vi "4 DDS 16SPC.vi"(8 "input valid":bool=TRUE, 9 "pdw in":T2 {"frequency shift" format="%#_12f"}, 10 "free DDS before me?":bool, 11 "new PDW in":bool) -> (0 "output valid":bool, 1 "state of every DDS":bool[](array[boolean]), 2 "have free DDS":bool, 3 "IQ out":T1[](array[typedef]))   [LabVIEW 2022 SP3]
doc: "transmit pulse with one free DDS inside.\nmust have no DDS before him (the distribute is to give the lowest mun DDS the pulse)"
uses:
  pulse_tx_vis/pdw.ctl
  pulse_tx_vis/mode_type.ctl
  <instrlib>/_niInstr/DSP/v1/Shared/Public/IQ Data.ctl
  <instrlib>/_niInstr/DSP/v1/Shared/niInstr DSP v1 Shared.lvlib
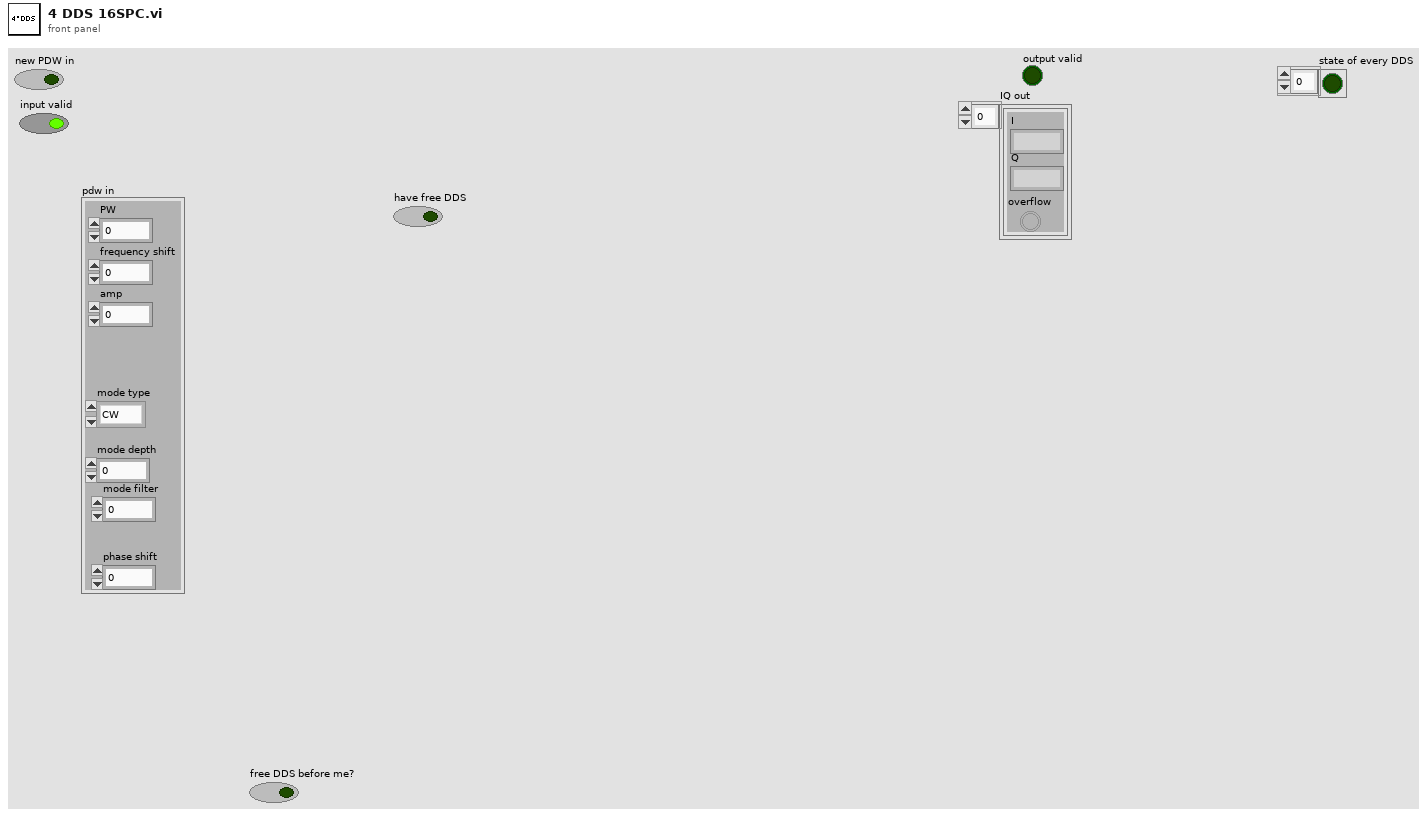
[diagram p1: front panel]
types:
  T1 = typedef "niInstr DSP v1 Shared.lvlib/IQ Data.ctl" = cluster{"I":fxp<+/-,18,1>, "Q":fxp<+/-,18,1>, "overflow":bool}
  T2 = typedef "pdw.ctl" = cluster{"PW":u32, "frequency shift":fxp<+/-,48,0>, "amp":fxp<+/-,18,1>, "mode type":T3, "mode depth":u32, "mode filter":u8, "phase shift":fxp<+/-,16,1>}
  T3 = typedef "mode_type.ctl" = enum8{"CW", "NC - CW", "NC - cw", "LFM", "BPSK", "QPSK"}
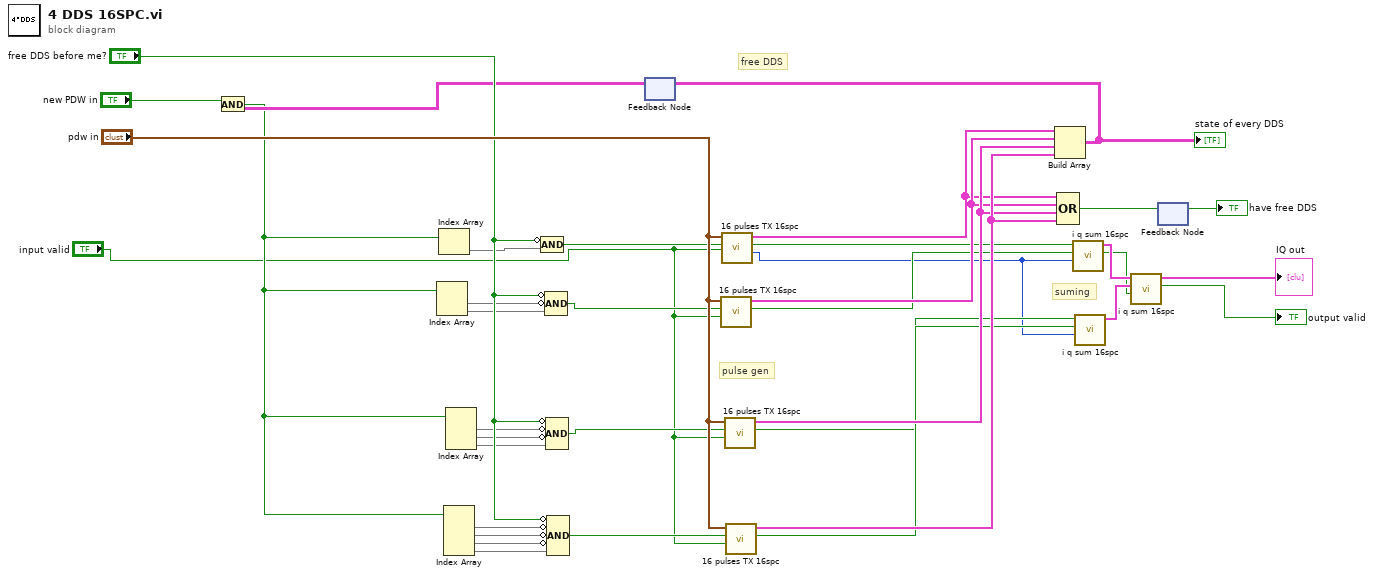
[diagram p0: block diagram]
diagram:
  # "free DDS"
  # "suming"
  # "pulse gen"
  n1 = feedback #1() -> (w9:T1[][])  [unwired: 1 in]
  n2 = And(x="new PDW in", y=w9) -> (x .and. y?=w8:bool)
  n3 = Index Array(array=w8) -> (element #1=w22, element #2=w20)  [unwired: 2 in]
  n4 = Index Array(array=w8) -> (element=w18)  [unwired: 1 in]
  n5 = Index Array(array=w8) -> (element #1=w30, element #2=w29, element #3=w28, element #4=w27)  [unwired: 4 in]
  n6 = Index Array(array=w8) -> (element #1=w26, element #2=w25, element #3=w24)  [unwired: 3 in]
  n7 = Compound Arithmetic op=AND(invert "free DDS before me?", w18) -> (w19:bool)
  n8 = Compound Arithmetic op=AND(invert "free DDS before me?", invert w22, w20) -> (w21:bool)
  n9 = Compound Arithmetic op=AND(invert "free DDS before me?", invert w26, invert w25, w24) -> (w23:bool)
  n10 = Compound Arithmetic op=AND(invert "free DDS before me?", invert w30, invert w29, invert w28, w27) -> (w31:bool)
  n11 = call "16 pulses TX 16spc.vi"("IQ_run"="input valid", "PDW input Valid"=w21, "array PDW"="pdw in") -> ("output valid"=w15:bool, "IQ out"=w33:T1[])  [unwired: 3 in, 4 out]
  n12 = call "16 pulses TX 16spc.vi"("IQ_run"="input valid", "PDW input Valid"=w19, "array PDW"="pdw in") -> ("fpga clock"=w4:u64, "output valid"=w14:bool, "IQ out"=w32:T1[])  [unwired: 3 in, 3 out]
  n13 = call "16 pulses TX 16spc.vi"("IQ_run"="input valid", "PDW input Valid"=w23, "array PDW"="pdw in") -> ("output valid"=w16:bool, "IQ out"=w34:T1[])  [unwired: 3 in, 4 out]
  n14 = call "16 pulses TX 16spc.vi"("IQ_run"="input valid", "PDW input Valid"=w31, "array PDW"="pdw in") -> ("output valid"=w17:bool, "IQ out"=w35:T1[])  [unwired: 3 in, 4 out]
  n15 = Build Array(w32, w33, w34, w35) -> (w11:T1[][])
  "state of every DDS" <- w11
  n16 = feedback-in #1(w11) -> ()
  n17 = Compound Arithmetic op=OR(w32, w33, w34, w35) -> (w7:bool)
  n18 = call "i q sum 16spc.vi"("input valid"=w4, "IQ in 2"=w15, "IQ in"=w14) -> ("output valid"=w3:bool, "IQ out"=w13:T1[])  [unwired: 7 in]
  n19 = call "i q sum 16spc.vi"("input valid"=w4, "IQ in 2"=w17, "IQ in"=w16) -> ("IQ out"=w12:T1[])  [unwired: 7 in, 1 out]
  n20 = call "i q sum 16spc.vi"("input valid"=w3, "IQ in 2"=w12, "IQ in"=w13) -> ("output valid"=→"output valid":bool, "IQ out"=→"IQ out":T1[])  [unwired: 7 in]
  n21 = feedback #2() -> (→"have free DDS":bool)  [unwired: 1 in]
  n22 = feedback-in #2(w7) -> ()
